vi "throttlecontroller2.vi"(11 "Boolean":bool=TRUE) -> ()   [LabVIEW 2015]
uses:
  RIOGlobal.vi
panel:
  out "sat":dbl
  out "Waveform Chart":dynamicdata(graph)
  out "P_GAIN":dbl=0.35
  in  "dead zone":dbl
  out "VS_TCU":dbl=20.125
  out "TPS":dbl=6.572769953051643
  out "VS_Desire":dbl=30.0
  out "T PWM":i16=2173
  in  "friction":dbl=500.0
  in  "step_size":dbl=0.05
  in  "derivative_gain":dbl=1.0
  in  "throttle_mapping":dbl=1.5
  in  "throttle_d_gain":dbl=0.4
  in  "gain_gain":dbl=0.1
  in  "gain":dbl=0.05
  in  "gain 1":dbl=700.0
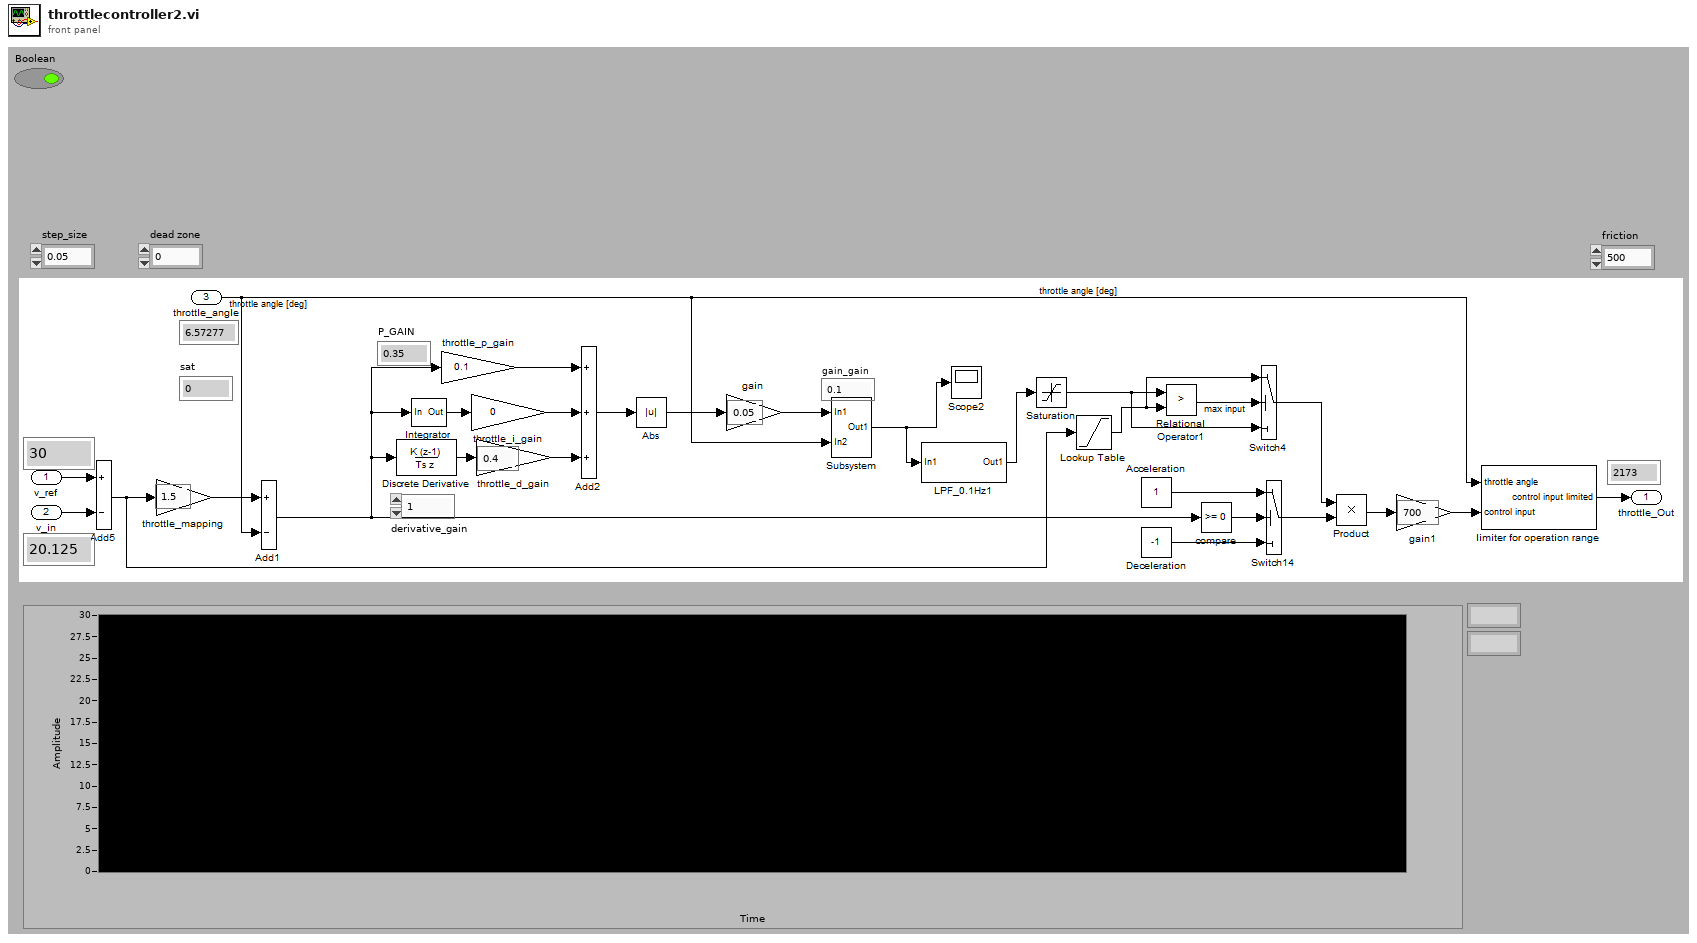
[diagram p1: front panel]
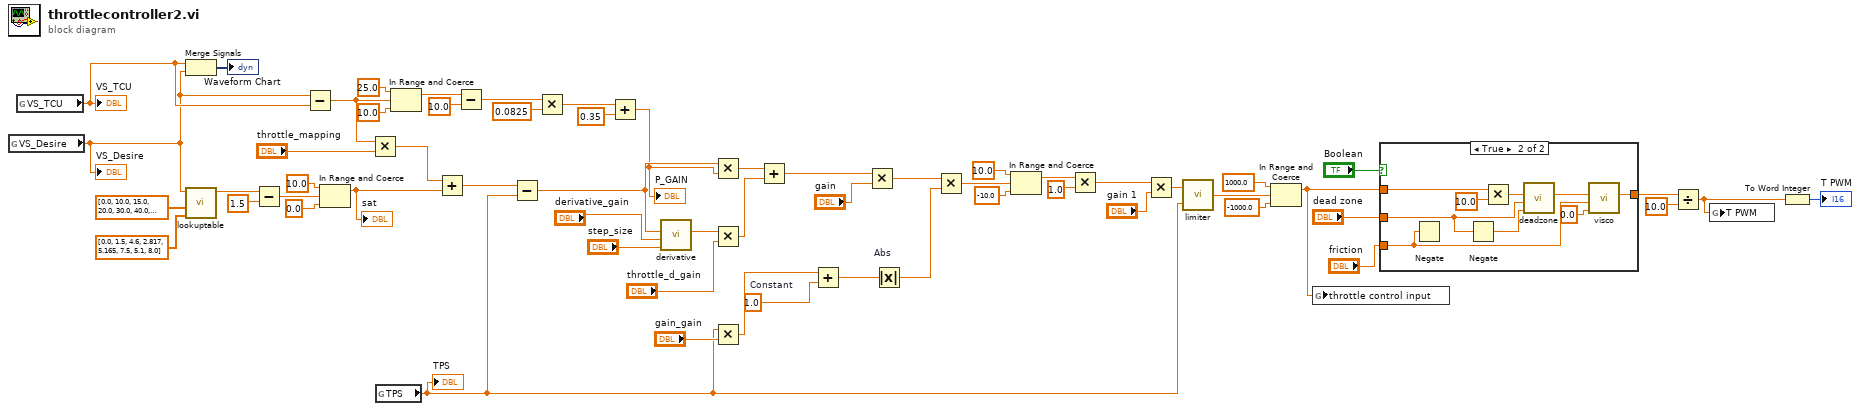
[diagram p0: block diagram]
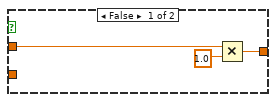
[diagram p2: hidden frame]
diagram:
  w59 = 1.0  # Constant
  n1 = global read "RIOGlobal.vi" "VS_Desire"() -> (w22:dbl)
  "VS_Desire" <- w22
  n2 = global read "RIOGlobal.vi" "VS_TCU"() -> (w24:dbl)
  "VS_TCU" <- w24
  n3 = Merge Signals(w24, w22) -> (→"Waveform Chart":dynamicdata)
  n4 = call "lookuptable.vi"("array_y"=dbl[] [0.0, 1.5, 4.6, 2.817, 5.165, 7.5, 5.1, 8.0] ("array_x"), "array_x"=dbl[] [0.0, 10.0, 15.0, 20.0, 30.0, 40.0, 50.0, 60.0], "x"=w22) -> ("y"=w20:dbl)  [unwired: 8 in]
  n5 = Subtract(x=w20, y=1.5) -> (x-y=w14:dbl)
  n6 = Subtract(x=w22, y=w24) -> (x-y=w10:dbl)
  n7 = In Range and Coerce(upper limit=10.0 ("max"), x=w14, lower limit=0.0 ("min")) -> (coerced(x)=w13:dbl)  [unwired: 1 out]
  "sat" <- w13
  n8 = Multiply(x=w10, y="throttle_mapping") -> (x*y=w18:dbl)
  n9 = global read "RIOGlobal.vi" "TPS"() -> (w37:dbl)
  "TPS" <- w37
  n10 = In Range and Coerce(upper limit=25.0 ("max"), x=w10, lower limit=10.0 ("min")) -> (coerced(x)=w9:dbl)  [unwired: 1 out]
  n11 = Add(x=w18, y=w13) -> (x+y=w17:dbl)
  n12 = Subtract(x=w9, y=10.0) -> (x-y=w32:dbl)
  n13 = Subtract(x=w17, y=w37) -> (x-y=w35:dbl)
  n14 = Multiply(x=w32, y=0.0825) -> (x*y=w31:dbl)
  n15 = Add(x=w31, y=0.35) -> (x+y=w29:dbl)
  "P_GAIN" <- w29
  n16 = call "derivative.vi"("step_size"="step_size", "gain"="derivative_gain", "input"=w35) -> ("output"=w46:dbl)  [unwired: 8 in]
  n17 = Multiply(x=w35, y=w29) -> (x*y=w48:dbl)
  n18 = Multiply(x=w46, y="throttle_d_gain") -> (x*y=w49:dbl)
  n19 = Multiply(x=w37, y="gain_gain") -> (x*y=w51:dbl)
  n20 = Add(x=w48, y=w49) -> (x+y=w39:dbl)
  n21 = Add(x=w51, y=w59) -> (x+y=w57:dbl)
  n22 = Multiply(x=w39, y="gain") -> (x*y=w53:dbl)
  n23 = Absolute Value "Abs"(x=w57) -> (abs(x)=w58:dbl)
  n24 = Multiply(x=w53, y=w58) -> (x*y=w8:dbl)
  n25 = In Range and Coerce(upper limit=10.0 ("max"), x=w8, lower limit=-10.0 ("min")) -> (coerced(x)=w5:dbl)  [unwired: 1 out]
  n26 = Multiply(x=w5, y=1.0) -> (x*y=w56:dbl)
  n27 = Multiply(x=w56, y="gain 1") -> (x*y=w43:dbl)
  n28 = call "limiter.vi"("throttle angle"=w37, "control input"=w43) -> ("control input limited"=w4:dbl)  [unwired: 1 in]
  n29 = In Range and Coerce(upper limit=1000.0 ("max"), x=w4, lower limit=-1000.0 ("min")) -> (coerced(x)=w1:dbl)  [unwired: 1 out]
  n30 = global write "RIOGlobal.vi" "throttle control input"(w1) -> ()
  n31 = case shown="True" "Boolean" {
    tunnel: [w60 w70] -> w28
    tunnel: "friction" -> [_ w69]
    tunnel: "dead zone" -> [_ w66]
    tunnel: w1 -> [w61 w65]
    frame False {
      n32 = Multiply(x=w61, y=1.0) -> (x*y=w60:dbl)
    }
    frame True {
      n33 = Negate(x=w69) -> ()  [unwired: 1 out]
      n34 = Negate(x=w66) -> (-x=w64:dbl)
      n35 = Multiply(x=w65, y=10.0) -> (x*y=w67:dbl)
      n36 = call "deadzone.vi"("min"=w64, "max"=w66, "x"=w67) -> ("dead zone"=w68:dbl)  [unwired: 8 in]
      n37 = call "visco.vi"("min"=0.0, "max"=w69, "input"=w68) -> ("output"=w70:dbl)  [unwired: 8 in]
    }
  }
  n38 = Divide(x=w28, y=10.0) -> (x/y=w26:dbl)
  n39 = global write "RIOGlobal.vi" "T PWM"(w26) -> ()
  n40 = To Word Integer(number=w26) -> (16bit integer=→"T PWM":i16)
